vi "Set One LED.vi"(8 "error in (no error)":errorcluster, 9 "Value":bool, 10 "Wash Step":T1, 11 "Simulated Wash Display Console in":refnum<class "Simulated Wash Display Console.lvclass">) -> (0 "error out":errorcluster, 3 "Simulated Wash Display Console out":refnum<class "Simulated Wash Display Console.lvclass">)   [LabVIEW 2012, in "Simulated Wash Display Console.lvlib" / "Simulated Wash Display Console.lvclass"]
uses:
  Simulated Wash Display Console.lvclass
  Car Wash Controller/Car Wash Controller/Wash Step.ctl
  Car Wash Controller/Car Wash Controller/Car Wash Controller.lvclass
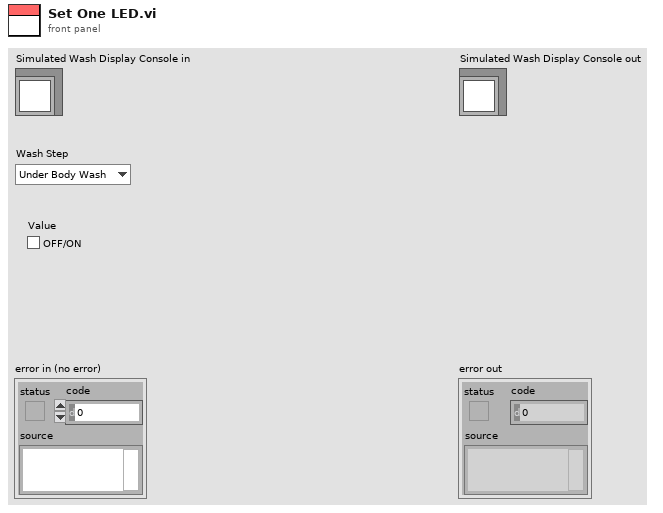
[diagram p1: front panel]
types:
  T1 = typedef "Car Wash Controller.lvlib/Car Wash Controller.lvclass/Wash Step.ctl" = enum16{"Under Body Wash", "Bug Remover", "Pre-Soak", "High Pressure Wash", "Low Pressure Wax", "Spot Free Rince", "Tire Shine Foam", "Air Dry"}
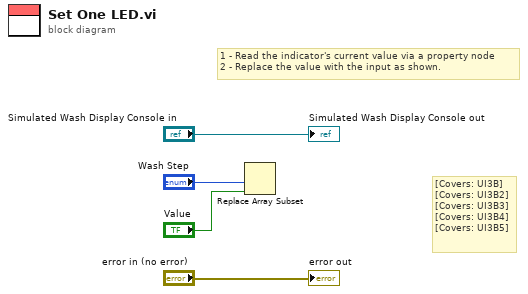
[diagram p0: block diagram]
diagram:
  # "[Covers: UI3B]\n[Covers: UI3B2]\n[Covers: UI3B3]\n[Covers: UI3B4]\n[Covers: UI3B5]"
  # "1 - Read the indicator's current value via a property node\n2 - Replace the value with the input as shown."
  n1 = Replace Array Subset(new element="Value", index="Wash Step") -> ()  [unwired: 1 in, 1 out]
  "error out" <- "error in (no error)"
  "Simulated Wash Display Console out" <- "Simulated Wash Display Console in"
